vi "GetBox.vi"(8 "error in (no error)":errorcluster, 11 "path to a png image":path) -> (0 "error out":errorcluster, 1 "edges coordinates":cluster{u32, u32, u32, u32})   [LabVIEW 2022 SP3]
doc: "This VI finds the coordinates for the edges of the pool table (png image).\n\nIt uses a double for-loop to find dark blue pixels which represent the borders of the table.\n\n--/!\\-- WARNING --/!\\-- \n\nThis VI uses a predefined RGB range to detect dark blue pixels :\n\nR : [0...24]\nG: [0...49]\nB : [100...119]\n\n--/!\\-- WARNING --/!\\-- \n\nInputs :\n- The path to png image\n- Error in\n\nOutputs :\n- A cluster containing Lmin, Lmax, Hmin and Hmax (in this order)\n- Error out"
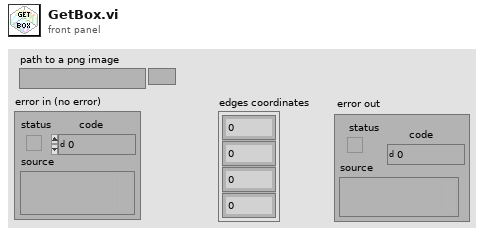
[diagram p1: front panel]
types:
  T1 = typedef "imagedata.ctl" = cluster{"image type":i32, "image depth":i32, "image":u8[], "mask":u8[], "colors":u32[], "Rectangle":cluster{"left":i16, "top":i16, "right":i16, "bottom":i16}}
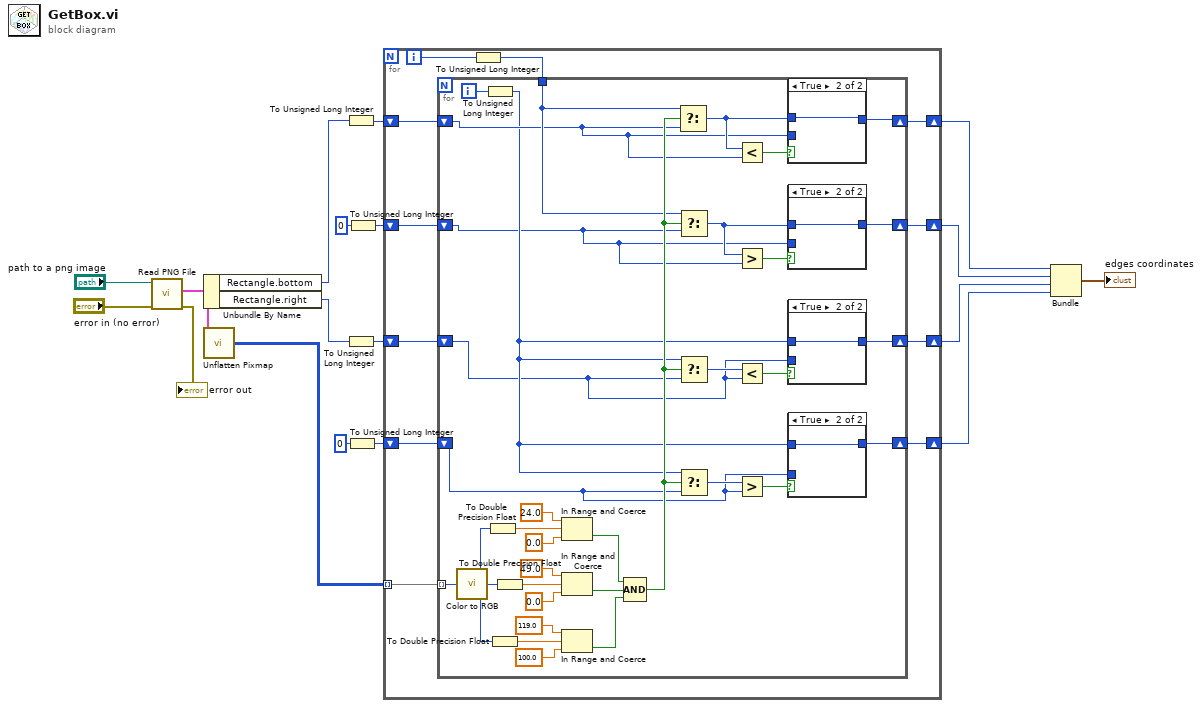
[diagram p0: block diagram]
diagram:
  n1 = call <vilib>:"Read PNG File.vi"("error in (no error)"="error in (no error)", "path to PNG file"="path to a png image") -> ("error out"=→"error out":errorcluster, "image data"=w18:T1)  [unwired: 7 in, 1 out]
  n2 = Unbundle By Name(w18) -> ("Rectangle.bottom"=w4:i16, "Rectangle.right"=w3:i16)
  n3 = call <vilib>:"Unflatten Pixmap.vi"("image data"=w18) -> ("24-bit pixmap"=w16:u32[][])  [unwired: 4 in, 6 out]
  n4 = To Unsigned Long Integer(number=w4) -> (unsigned 32bit integer=w12:u32)
  n5 = To Unsigned Long Integer(number=w3) -> (unsigned 32bit integer=w13:u32)
  n6 = To Unsigned Long Integer(number=0) -> (unsigned 32bit integer=w11:u32)
  n7 = To Unsigned Long Integer(number=0) -> (unsigned 32bit integer=w10:u32)
  n8 = for {
    tunnel: w16 -> [w29] mode=indexing
    shift-right: [w28] -> w5
    shift-left: w13 -> [w24]
    shift-right: [w26] -> w6
    shift-left: w11 -> [w22]
    shift-right: [w25] -> w9
    shift-left: w12 -> [w21]
    shift-right: [w27] -> w7
    shift-left: w10 -> [w23]
    i -> [w20]
    n9 = To Unsigned Long Integer(number=w20) -> (unsigned 32bit integer=w19:u32)
    n10 = for {
      tunnel: w29 -> [w65] mode=indexing
      shift-right: [w46] -> w26
      shift-left: w22 -> [w36]
      shift-right: [w48] -> w28
      shift-left: w24 -> [w37]
      shift-right: [w45] -> w25
      shift-left: w21 -> [w40]
      shift-right: [w47] -> w27
      shift-left: w23 -> [w38]
      tunnel: w19 -> [w41]
      i -> [w43]
      n11 = call <vilib>:"Color to RGB.vi"("Color"=w65) -> ("R"=w62:u8, "G"=w63:u8, "B"=w64:u8)  [unwired: 1 out]
      n12 = To Unsigned Long Integer(number=w43) -> (unsigned 32bit integer=w39:u32)
      n13 = To Double Precision Float(number=w62) -> (double precision float=w61:dbl)
      n14 = To Double Precision Float(number=w64) -> (double precision float=w59:dbl)
      n15 = To Double Precision Float(number=w63) -> (double precision float=w60:dbl)
      n16 = In Range and Coerce(upper limit=24.0, x=w61, lower limit=0.0) -> (In Range?=w56:bool)  [unwired: 1 out]
      n17 = In Range and Coerce(upper limit=49.0, x=w60, lower limit=0.0) -> (In Range?=w57:bool)  [unwired: 1 out]
      n18 = In Range and Coerce(upper limit=119.0, x=w59, lower limit=100.0) -> (In Range?=w58:bool)  [unwired: 1 out]
      n19 = Compound Arithmetic op=AND(w56, w57, w58) -> (w55:bool)
      n20 = Select(t=w41, s=w55, f=w40) -> (s? t:f=w42:u32)
      n21 = Select(t=w41, s=w55, f=w38) -> (s? t:f=w44:u32)
      n22 = Select(t=w39, s=w55, f=w37) -> (s? t:f=w53:u32)
      n23 = Select(t=w39, s=w55, f=w36) -> (s? t:f=w54:u32)
      n24 = Less?(x=w42, y=w40) -> (x < y?=w50:bool)
      n25 = Greater?(x=w44, y=w38) -> (0:w52:bool)
      n26 = Less?(x=w53, y=w37) -> (x < y?=w49:bool)
      n27 = Greater?(x=w54, y=w36) -> (0:w51:bool)
      n28 = case shown="True" w50 {
        tunnel: [w72 w73] -> w45
        tunnel: w40 -> [w72 _]
        tunnel: w42 -> [_ w73]
        frame False {
        }
        frame True {
        }
      }
      n29 = case shown="True" w52 {
        tunnel: [w68 w69] -> w47
        tunnel: w44 -> [_ w69]
        tunnel: w38 -> [w68 _]
        frame False {
        }
        frame True {
        }
      }
      n30 = case shown="True" w49 {
        tunnel: [w66 w67] -> w48
        tunnel: w39 -> [_ w67]
        tunnel: w37 -> [w66 _]
        frame False {
        }
        frame True {
        }
      }
      n31 = case shown="True" w51 {
        tunnel: [w70 w71] -> w46
        tunnel: w39 -> [_ w71]
        tunnel: w36 -> [w70 _]
        frame False {
        }
        frame True {
        }
      }
    }
  }
  n32 = Bundle(w9, w7, w5, w6) -> (→"edges coordinates":cluster{u32, u32, u32, u32})  [unwired: 1 in]
